vi "MCB2400 AI Scan Specify Node.vi"(10 "Node Attributes":T2, 11 "Attributes":T1 {"Programmable Pin Connections" items=["AI Bank uses AI channels 0-7, which use pins P0.12, P0.13, P0.23, P0.24, P0.25, P0.26, P1.30, and P1.31. You cannot use AI Bank and AI0-7 or these pins in the same project."]}) -> (3 "type out":T3)   [LabVIEW 2011]
doc: "This VI is a \"Specify Node\" vi. It is used to pick which I/O Implementation VI to use when more than one is specified for an I/O resource. This VI looks at the Node Attributes and selects the type of the I/O based on whether the user selects array or scalar data and whether they select scaled or raw binary. The output is a variant that indicates the type returned by the I/O and it must match the type of one of the I/O Implementation VIs."
uses:
  <vilib>/eio/EIO_TypeDescriptor.ctl
  <vilib>/Embedded/ARM/MCB2400/MCB2400_AI_Scan_NodeAttr.ctl
  <vilib>/Embedded/ARM/MCB2400/MCB2400_AI_Scan_PrjAttr.ctl
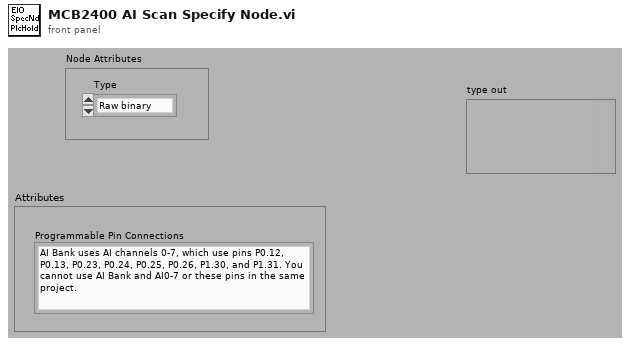
[diagram p1: front panel]
types:
  T1 = typedef "MCB2400_AI_Scan_PrjAttr.ctl" = cluster{"Programmable Pin Connections":u16}
  T2 = typedef "MCB2400_AI_Scan_NodeAttr.ctl" = cluster{"Type":enum16{"Raw binary", "Scaled voltage"}}
  T3 = typedef "EIO_TypeDescriptor.ctl" = variant
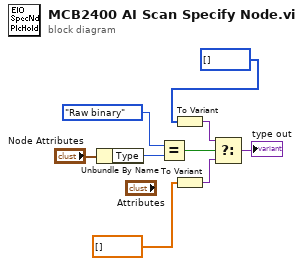
[diagram p0: block diagram]
diagram:
  n1 = Unbundle By Name("Node Attributes") -> ("Type"=w5:enum16{"Raw binary", "Scaled voltage"})
  n2 = Equal?(x=enum16{"Raw binary", "Scaled voltage"}."Raw binary" ("Type"), y=w5) -> (x = y?=w4:bool)
  n3 = To Variant(anything=i32[] []) -> (Variant=w7:variant)
  n4 = To Variant(anything=dbl[] []) -> (Variant=w8:variant)
  n5 = Select(t=w7, s=w4, f=w8) -> (s? t:f=→"type out":variant)
